vi "FL_Decode_RAW_to_DEC_bit_split.vi"(1 "Input timestamp":timestamp, 2 "Read buffer text to decode":string, 3 "Sensor board size":string="Small") -> (0 "DEC output cluster":T1)   [LabVIEW 2016]
panel:
  in  "X off Large":sgl=-1.0
  in  "Y off Large":sgl=3.0
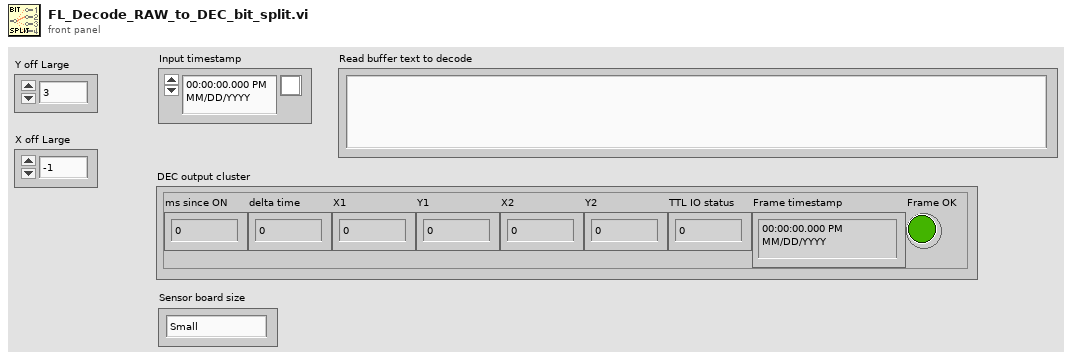
[diagram p1: front panel]
types:
  T1 = cluster{"ms since ON":u32, "delta time":u32, "X1":sgl, "Y1":sgl, "X2":sgl, "Y2":sgl, "TTL IO status":u8, "Frame timestamp":timestamp, "Frame OK":bool}
  T2 = cluster{"Half-width of the sensor board":sgl, "Half-height of the sensor board":sgl, "Sensors grid step":sgl}
  T3 = cluster{u32, u32, sgl, sgl, sgl, sgl, u8, "Input timestamp":timestamp, bool}
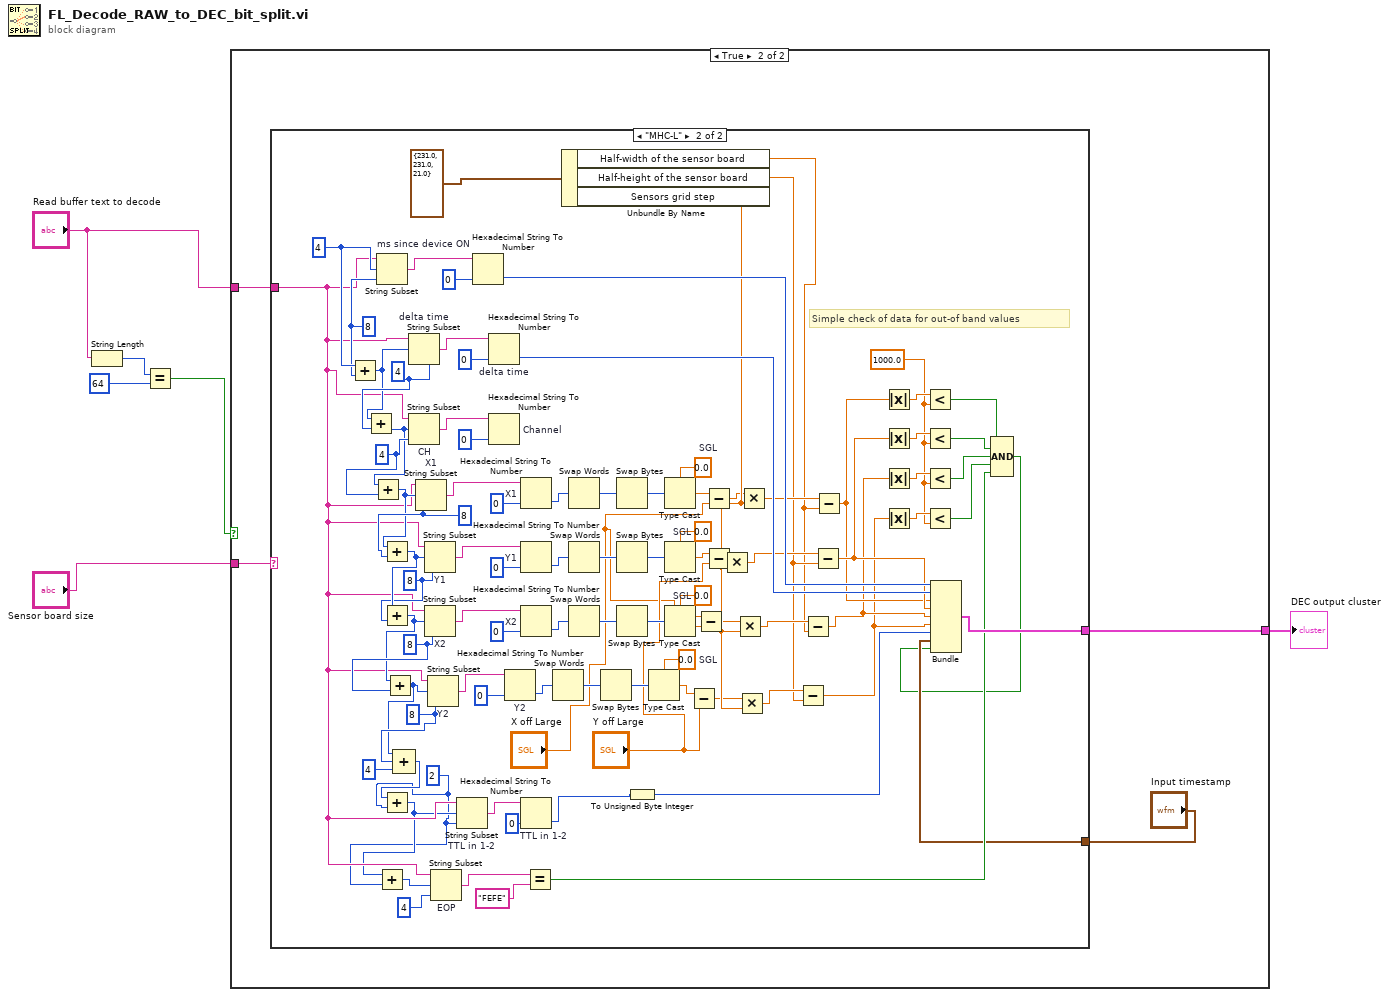
[diagram p0: block diagram]
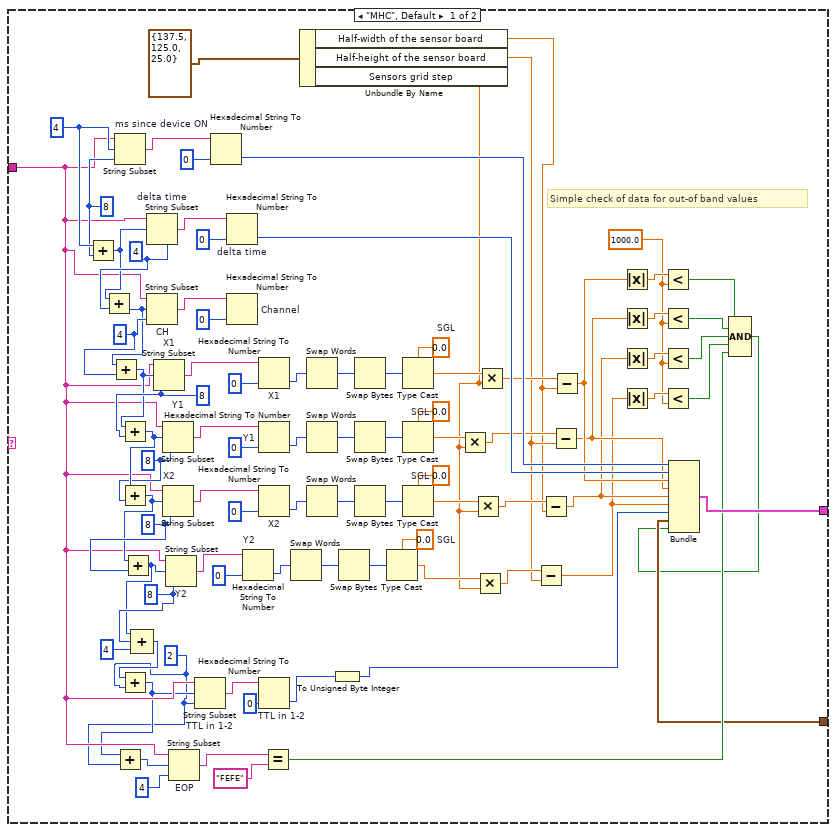
[diagram p3: hidden frame]
diagram:
  n1 = String Length(string="Read buffer text to decode") -> (length=w4:i32)
  n2 = Equal?(x=w4, y=64) -> (x = y?=w2:bool)
  n3 = case shown="True" w2 {
    tunnel: [_ w10] -> w6
    tunnel: "Read buffer text to decode" -> [_ w9]
    tunnel: "Sensor board size" -> [_ w8]
    frame False {
    }
    frame True {
      n4 = case shown="\"MHC-L\"" w8 {
        tunnel: [w40 w138] -> w10
        tunnel: w9 -> [w37 w135]
        tunnel: "Input timestamp" -> [w12 w110]
        frame "MHC", Default {
          w24 = 1000.0
          w96 = 4
          w35 = 2 ("length (rest)")
          w82 = sgl 0.0  # SGL
          w75 = sgl 0.0  # SGL
          w68 = sgl 0.0  # SGL
          w62 = sgl 0.0  # SGL
          w91 = 8 ("length (rest)")
          w51 = 8 ("length (rest)")
          w48 = 8 ("length (rest)")
          w47 = 8 ("length (rest)")
          w45 = 4 ("length (rest)")
          w43 = 4 ("length (rest)")
          w41 = 8 ("length (rest)")
          # "Simple check of data for out-of band values"
          n5 = Add(x=w96, y=w41) -> (x+y=w42:i32)
          n6 = Add(x=w42, y=w43) -> (x+y=w44:i32)
          n7 = Add(x=w44, y=w45) -> (x+y=w46:i32)
          n8 = String Subset "ms since device ON"(string=w37, offset (0)=w96, length (rest)=w41) -> (substring=w52:string)
          n9 = Add(x=w46, y=w47) -> (x+y=w49:i32)
          n10 = Add(x=w49, y=w48) -> (x+y=w50:i32)
          n11 = Add(x=w50, y=w51) -> (x+y=w90:i32)
          n12 = Compound Arithmetic op=unknown(w90, w91, 4 ("value")) -> (w94:i32)
          n13 = Add(x=w94, y=w35) -> (x+y=w36:i32)
          n14 = Add(x=w36, y=w35) -> (x+y=w39:i32)
          n15 = String Subset "delta time"(string=w37, offset (0)=w42, length (rest)=w43) -> (substring=w55:string)
          n16 = String Subset "CH"(string=w37, offset (0)=w44, length (rest)=w45) -> (substring=w57:string)
          n17 = String Subset "X1"(string=w37, offset (0)=w46, length (rest)=w47) -> (substring=w58:string)
          n18 = String Subset "Y1"(string=w37, offset (0)=w49, length (rest)=w48) -> (substring=w70:string)
          n19 = String Subset "X2"(string=w37, offset (0)=w50, length (rest)=w51) -> (substring=w77:string)
          n20 = String Subset "Y2"(string=w37, offset (0)=w90, length (rest)=w91) -> (substring=w84:string)
          n21 = String Subset "EOP"(string=w37, offset (0)=w39, length (rest)=4 ("length (rest)")) -> (substring=w34:string)
          n22 = String Subset "TTL in 1-2"(string=w37, offset (0)=w36, length (rest)=w35) -> (substring=w92:string)
          n23 = Hexadecimal String To Number ("ms since ON")(string=w52, default (0uL)=u32 0 ("default (0 U32)")) -> (number=w98:u32)  [unwired: 1 in, 1 out]
          n24 = Hexadecimal String To Number "delta time"(string=w55, default (0uL)=u32 0 ("default (0 U32)")) -> (number=w97:u32)  [unwired: 1 in, 1 out]
          n25 = Hexadecimal String To Number "Channel"(string=w57, default (0uL)=u32 0 ("default (0 U32)")) -> ()  [unwired: 1 in, 2 out]
          n26 = Hexadecimal String To Number "Y2"(string=w84, default (0uL)=u32 0 ("default (0 U32)")) -> (number=w80:u32)  [unwired: 1 in, 1 out]
          n27 = Hexadecimal String To Number "X1"(string=w58, default (0uL)=u32 0 ("default (0 U32)")) -> (number=w60:u32)  [unwired: 1 in, 1 out]
          n28 = Hexadecimal String To Number "Y1"(string=w70, default (0uL)=u32 0 ("default (0 U32)")) -> (number=w66:u32)  [unwired: 1 in, 1 out]
          n29 = Hexadecimal String To Number "X2"(string=w77, default (0uL)=u32 0 ("default (0 U32)")) -> (number=w73:u32)  [unwired: 1 in, 1 out]
          n30 = Hexadecimal String To Number "TTL in 1-2"(string=w92, default (0uL)=u32 0 ("default (0 U32)")) -> (number=w14:u32)  [unwired: 1 in, 1 out]
          n31 = Equal?(x=w34, y="FEFE") -> (x = y?=w19:bool)
          n32 = Swap Words(1:w80) -> (0:w81:u32)
          n33 = Unbundle By Name(T2 {"Half-width of the sensor board"=137.5, "Half-height of the sensor board"=125.0, "Sensors grid step"=25.0} ("MHC geometry")) -> ("Half-width of the sensor board"=w16:sgl, "Half-height of the sensor board"=w17:sgl, "Sensors grid step"=w18:sgl)
          n34 = Swap Words(1:w60) -> (0:w61:u32)
          n35 = Swap Words(1:w66) -> (0:w67:u32)
          n36 = Swap Words(1:w73) -> (0:w74:u32)
          n37 = To Unsigned Byte Integer(number=w14) -> (unsigned 8bit integer=w13:u8)
          n38 = Swap Bytes(anything=w81) -> (byte swapped=w83:u32)
          n39 = Swap Bytes(anything=w61) -> (byte swapped=w63:u32)
          n40 = Swap Bytes(anything=w67) -> (byte swapped=w69:u32)
          n41 = Swap Bytes(anything=w74) -> (byte swapped=w76:u32)
          n42 = Type Cast(type=w82, x=w83) -> (*(type *) &x=w85:sgl)
          n43 = Type Cast(type=w62, x=w63) -> (*(type *) &x=w64:sgl)
          n44 = Type Cast(type=w68, x=w69) -> (*(type *) &x=w71:sgl)
          n45 = Type Cast(type=w75, x=w76) -> (*(type *) &x=w78:sgl)
          n46 = Multiply(x=w71, y=w18) -> (x*y=w88:sgl)
          n47 = Multiply(x=w78, y=w18) -> (x*y=w87:sgl)
          n48 = Multiply(x=w85, y=w18) -> (x*y=w89:sgl)
          n49 = Multiply(x=w64, y=w18) -> (x*y=w86:sgl)
          n50 = Subtract(x=w89, y=w17) -> (x-y=w29:sgl)
          n51 = Subtract(x=w87, y=w16) -> (x-y=w30:sgl)
          n52 = Subtract(x=w88, y=w17) -> (x-y=w31:sgl)
          n53 = Subtract(x=w86, y=w16) -> (x-y=w32:sgl)
          n54 = Absolute Value(x=w32) -> (abs(x)=w28:sgl)
          n55 = Absolute Value(x=w31) -> (abs(x)=w26:sgl)
          n56 = Absolute Value(x=w30) -> (abs(x)=w27:sgl)
          n57 = Absolute Value(x=w29) -> (abs(x)=w25:sgl)
          n58 = Less?(x=w28, y=w24) -> (x < y?=w23:bool)
          n59 = Less?(x=w26, y=w24) -> (x < y?=w22:bool)
          n60 = Less?(x=w27, y=w24) -> (x < y?=w21:bool)
          n61 = Less?(x=w25, y=w24) -> (x < y?=w20:bool)
          n62 = Compound Arithmetic op=AND(w23, w22, w21, w20, w19) -> (w11:bool)
          n63 = Bundle(w98, w97, w32, w31, w30, w29, w13, "Input timestamp"=w12, w11) -> (w40:T3)  [unwired: 1 in]
        }
        frame "MHC-L" {
          w126 = 1000.0
          w190 = 4
          w133 = 2 ("length (rest)")
          w177 = sgl 0.0  # SGL
          w171 = sgl 0.0  # SGL
          w165 = sgl 0.0  # SGL
          w160 = sgl 0.0  # SGL
          w185 = 8 ("length (rest)")
          w149 = 8 ("length (rest)")
          w146 = 8 ("length (rest)")
          w145 = 8 ("length (rest)")
          w143 = 4 ("length (rest)")
          w141 = 4 ("length (rest)")
          w139 = 8 ("length (rest)")
          # "Simple check of data for out-of band values"
          n64 = Add(x=w190, y=w139) -> (x+y=w140:i32)
          n65 = Add(x=w140, y=w141) -> (x+y=w142:i32)
          n66 = Add(x=w142, y=w143) -> (x+y=w144:i32)
          n67 = String Subset "ms since device ON"(string=w135, offset (0)=w190, length (rest)=w139) -> (substring=w150:string)
          n68 = Add(x=w144, y=w145) -> (x+y=w147:i32)
          n69 = Add(x=w147, y=w146) -> (x+y=w148:i32)
          n70 = Add(x=w148, y=w149) -> (x+y=w184:i32)
          n71 = Compound Arithmetic op=unknown(w184, w185, 4 ("value")) -> (w188:i32)
          n72 = Add(x=w188, y=w133) -> (x+y=w134:i32)
          n73 = Add(x=w134, y=w133) -> (x+y=w137:i32)
          n74 = String Subset "delta time"(string=w135, offset (0)=w140, length (rest)=w141) -> (substring=w153:string)
          n75 = String Subset "CH"(string=w135, offset (0)=w142, length (rest)=w143) -> (substring=w155:string)
          n76 = String Subset "X1"(string=w135, offset (0)=w144, length (rest)=w145) -> (substring=w156:string)
          n77 = String Subset "Y1"(string=w135, offset (0)=w147, length (rest)=w146) -> (substring=w167:string)
          n78 = String Subset "X2"(string=w135, offset (0)=w148, length (rest)=w149) -> (substring=w173:string)
          n79 = String Subset "Y2"(string=w135, offset (0)=w184, length (rest)=w185) -> (substring=w179:string)
          n80 = String Subset "EOP"(string=w135, offset (0)=w137, length (rest)=4 ("length (rest)")) -> (substring=w132:string)
          n81 = String Subset "TTL in 1-2"(string=w135, offset (0)=w134, length (rest)=w133) -> (substring=w186:string)
          n82 = Hexadecimal String To Number ("ms since ON")(string=w150, default (0uL)=u32 0 ("default (0 U32)")) -> (number=w192:u32)  [unwired: 1 in, 1 out]
          n83 = Hexadecimal String To Number "delta time"(string=w153, default (0uL)=u32 0 ("default (0 U32)")) -> (number=w191:u32)  [unwired: 1 in, 1 out]
          n84 = Hexadecimal String To Number "Channel"(string=w155, default (0uL)=u32 0 ("default (0 U32)")) -> ()  [unwired: 1 in, 2 out]
          n85 = Hexadecimal String To Number "Y2"(string=w179, default (0uL)=u32 0 ("default (0 U32)")) -> (number=w175:u32)  [unwired: 1 in, 1 out]
          n86 = Hexadecimal String To Number "X1"(string=w156, default (0uL)=u32 0 ("default (0 U32)")) -> (number=w158:u32)  [unwired: 1 in, 1 out]
          n87 = Hexadecimal String To Number "Y1"(string=w167, default (0uL)=u32 0 ("default (0 U32)")) -> (number=w163:u32)  [unwired: 1 in, 1 out]
          n88 = Hexadecimal String To Number "X2"(string=w173, default (0uL)=u32 0 ("default (0 U32)")) -> (number=w169:u32)  [unwired: 1 in, 1 out]
          n89 = Hexadecimal String To Number "TTL in 1-2"(string=w186, default (0uL)=u32 0 ("default (0 U32)")) -> (number=w112:u32)  [unwired: 1 in, 1 out]
          n90 = Equal?(x=w132, y="FEFE") -> (x = y?=w121:bool)
          n91 = Swap Words(1:w175) -> (0:w176:u32)
          n92 = Unbundle By Name(T2 {"Half-width of the sensor board"=231.0, "Half-height of the sensor board"=231.0, "Sensors grid step"=21.0} ("MHC geometry")) -> ("Half-width of the sensor board"=w118:sgl, "Half-height of the sensor board"=w119:sgl, "Sensors grid step"=w120:sgl)
          n93 = Swap Words(1:w158) -> (0:w159:u32)
          n94 = Swap Words(1:w163) -> (0:w164:u32)
          n95 = Swap Words(1:w169) -> (0:w170:u32)
          n96 = Swap Bytes(anything=w176) -> (byte swapped=w178:u32)
          n97 = Swap Bytes(anything=w159) -> (byte swapped=w161:u32)
          n98 = Swap Bytes(anything=w164) -> (byte swapped=w166:u32)
          n99 = Swap Bytes(anything=w170) -> (byte swapped=w172:u32)
          n100 = To Unsigned Byte Integer(number=w112) -> (unsigned 8bit integer=w111:u8)
          n101 = Type Cast(type=w177, x=w178) -> (*(type *) &x=w101:sgl)
          n102 = Type Cast(type=w160, x=w161) -> (*(type *) &x=w104:sgl)
          n103 = Type Cast(type=w165, x=w166) -> (*(type *) &x=w103:sgl)
          n104 = Type Cast(type=w171, x=w172) -> (*(type *) &x=w102:sgl)
          n105 = Subtract(x=w101, y="Y off Large") -> (x-y=w113:sgl)
          n106 = Subtract(x=w102, y="X off Large") -> (x-y=w114:sgl)
          n107 = Subtract(x=w104, y="X off Large") -> (x-y=w116:sgl)
          n108 = Subtract(x=w103, y="Y off Large") -> (x-y=w115:sgl)
          n109 = Multiply(x=w115, y=w120) -> (x*y=w182:sgl)
          n110 = Multiply(x=w114, y=w120) -> (x*y=w181:sgl)
          n111 = Multiply(x=w113, y=w120) -> (x*y=w183:sgl)
          n112 = Multiply(x=w116, y=w120) -> (x*y=w180:sgl)
          n113 = Subtract(x=w183, y=w119) -> (x-y=w105:sgl)
          n114 = Subtract(x=w181, y=w118) -> (x-y=w106:sgl)
          n115 = Subtract(x=w182, y=w119) -> (x-y=w108:sgl)
          n116 = Subtract(x=w180, y=w118) -> (x-y=w107:sgl)
          n117 = Absolute Value(x=w107) -> (abs(x)=w130:sgl)
          n118 = Absolute Value(x=w108) -> (abs(x)=w128:sgl)
          n119 = Absolute Value(x=w106) -> (abs(x)=w129:sgl)
          n120 = Absolute Value(x=w105) -> (abs(x)=w127:sgl)
          n121 = Less?(x=w130, y=w126) -> (x < y?=w125:bool)
          n122 = Less?(x=w128, y=w126) -> (x < y?=w124:bool)
          n123 = Less?(x=w129, y=w126) -> (x < y?=w123:bool)
          n124 = Less?(x=w127, y=w126) -> (x < y?=w122:bool)
          n125 = Compound Arithmetic op=AND(w125, w124, w123, w122, w121) -> (w109:bool)
          n126 = Bundle(w192, w191, w107, w108, w106, w105, w111, "Input timestamp"=w110, w109) -> (w138:T3)  [unwired: 1 in]
        }
      }
    }
  }
  "DEC output cluster" <- w6
